vi "LJUD U3RAW Watchdog.vi"(4 "DIOConfig":u8, 6 "WriteMask":u8, 7 "Comm Settings":T1={"Open LabJack "=TRUE, "Address"="1", "FirstFound"=TRUE}, 8 "error in (no error)":errorcluster, 9 "TimeoutPeriod":u16=10, 10 "WatchdogOptions":u8, 11 "Handle In":i32) -> (0 "error out":errorcluster, 3 "Handle Out":i32)   [LabVIEW 2021]
panel:
  out "Read Array":u8[](array[numeric]) format="%.0x"
  # "Bit 0:  Write"
  # "WatchdogOptions:\nBit 5:  Reset\nBit 4:  Update Digital I/O"
  # "~Seconds"
  # "Bit 7:  State\nBit 4-0:  Digital I/O #"
  # "If open is false,\nthen a valid\nhandle must be\npassed in."
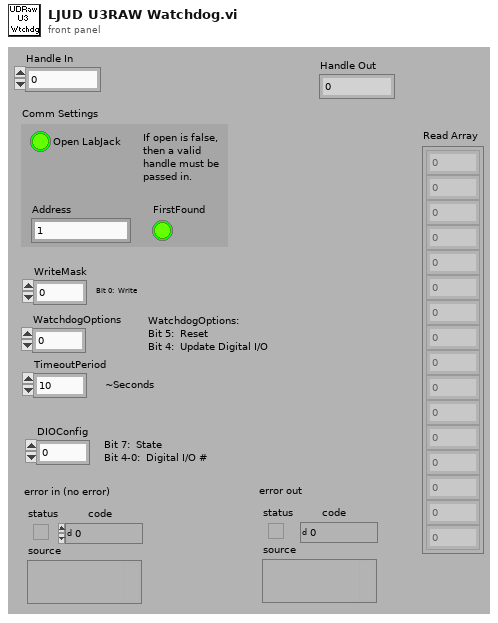
[diagram p1: front panel]
types:
  T1 = cluster{"Open LabJack ":bool, "Address":string, "FirstFound":bool}
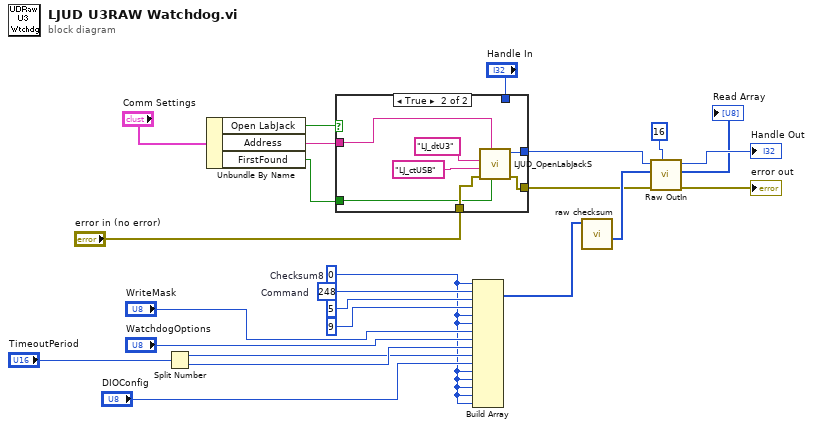
[diagram p0: block diagram]
diagram:
  w10 = u8 0  # Checksum8
  w24 = u8 248  # Command
  n1 = Split Number(x="TimeoutPeriod") -> (hi(x)=w18:u8, lo(x)=w19:u8)
  n2 = Unbundle By Name("Comm Settings") -> ("Open LabJack"=w8:bool, "Address"=w7:string, "FirstFound"=w6:bool)
  n3 = case shown="True" w8 {
    tunnel: w7 -> [_ w30]
    tunnel: "error in (no error)" -> [w26 w31]
    tunnel: [w26 w32] -> w4
    tunnel: [w25 w33] -> w3
    tunnel: w6 -> [_ w29]
    tunnel: "Handle In" -> [w25 _]
    frame False {
    }
    frame True {
      n4 = call "LJUD_OpenLabJackS.vi"("FirstFound"=w29, "Address"=w30, "error in"=w31, "ConnectionType"="LJ_ctUSB", "DeviceType"="LJ_dtU3") -> ("error out"=w32:errorcluster, "Handle"=w33:i32)  [unwired: 4 in, 1 out]
    }
  }
  n5 = Build Array(w10, w24, u8 5, u8 9, w10, w10, "WriteMask", "WatchdogOptions", w19, w18, "DIOConfig", w10, w10, w10, w10, w10) -> (w15:u8[])
  n6 = call "raw checksum.vi"("Array"=w15) -> ("Array Output"=w17:u8[])  [unwired: 3 in, 7 out]
  n7 = call "Raw OutIn.vi"("# of bytes to read in"=16 ("# of bytes to read"), "error in"=w4, "Raw Out"=w17, "Handle In"=w3) -> ("error out"=→"error out":errorcluster, "Raw In"=→"Read Array":u8[], "Handle Out"=→"Handle Out":i32)  [unwired: 4 in, 1 out]
